vi "LoadGCSLowLevelVIs.vi"(11 "GCS Merged Drivers Low-Level Path":path) -> (3 "PI GCS Function\nReferences":T1)   [LabVIEW 2011]
uses:
  GCS_Interface.ctl
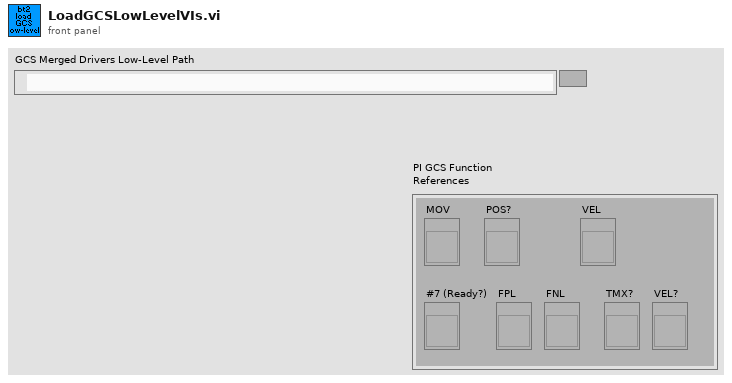
[diagram p1: front panel]
types:
  T1 = typedef "GCS_Interface.ctl" = cluster{"MOV":refnum<vi>, "VEL":refnum<vi>, "VEL?":refnum<vi>, "POS?":refnum<vi>, "TMX?":refnum<vi>, "#7 (Ready?)":refnum<vi>, "FPL":refnum<vi>, "FNL":refnum<vi>}
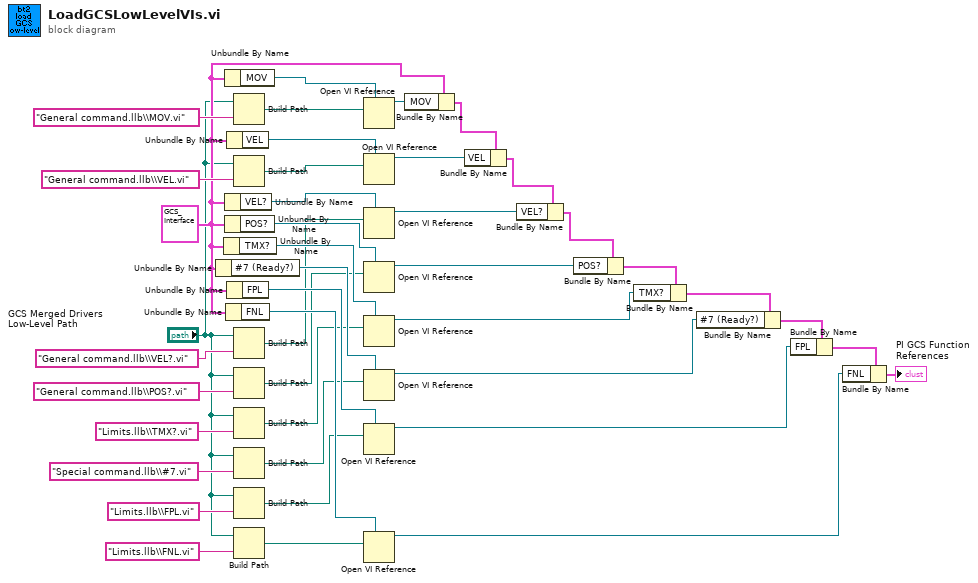
[diagram p0: block diagram]
diagram:
  w26 = T1 {"MOV"=refnum, "VEL"=refnum, "VEL?"=refnum, "POS?"=refnum, "TMX?"=refnum, "#7 (Ready?)"=refnum, "FPL"=refnum, "FNL"=refnum} ("PI GCS Function\nReferences")
  n1 = Unbundle By Name(w26) -> ("#7 (Ready?)"=w34:refnum<vi>)
  n2 = Unbundle By Name(w26) -> ("TMX?"=w37:refnum<vi>)
  n3 = Unbundle By Name(w26) -> ("MOV"=w33:refnum<vi>)
  n4 = Unbundle By Name(w26) -> ("VEL?"=w32:refnum<vi>)
  n5 = Unbundle By Name(w26) -> ("POS?"=w35:refnum<vi>)
  n6 = Unbundle By Name(w26) -> ("FNL"=w29:refnum<vi>)
  n7 = Unbundle By Name(w26) -> ("VEL"=w31:refnum<vi>)
  n8 = Unbundle By Name(w26) -> ("FPL"=w30:refnum<vi>)
  n9 = Build Path(base path="GCS Merged Drivers Low-Level Path", name or relative path="General command.llb\\MOV.vi") -> (appended path=w17:path)
  n10 = Build Path(base path="GCS Merged Drivers Low-Level Path", name or relative path="General command.llb\\VEL.vi") -> (appended path=w15:path)
  n11 = Build Path(base path="GCS Merged Drivers Low-Level Path", name or relative path="General command.llb\\VEL?.vi") -> (appended path=w12:path)
  n12 = Build Path(base path="GCS Merged Drivers Low-Level Path", name or relative path="General command.llb\\POS?.vi") -> (appended path=w27:path)
  n13 = Build Path(base path="GCS Merged Drivers Low-Level Path", name or relative path="Limits.llb\\TMX?.vi") -> (appended path=w10:path)
  n14 = Build Path(base path="GCS Merged Drivers Low-Level Path", name or relative path="Special command.llb\\#7.vi") -> (appended path=w5:path)
  n15 = Build Path(base path="GCS Merged Drivers Low-Level Path", name or relative path="Limits.llb\\FPL.vi") -> (appended path=w4:path)
  n16 = Build Path(base path="GCS Merged Drivers Low-Level Path", name or relative path="Limits.llb\\FNL.vi") -> (appended path=w1:path)
  n17 = Open VI Reference(type specifier VI Refnum (for type only)=w33, vi path=w17) -> (vi reference=w16:refnum<vi>)  [unwired: 4 in, 1 out]
  n18 = Open VI Reference(type specifier VI Refnum (for type only)=w31, vi path=w15) -> (vi reference=w14:refnum<vi>)  [unwired: 4 in, 1 out]
  n19 = Open VI Reference(type specifier VI Refnum (for type only)=w32, vi path=w12) -> (vi reference=w13:refnum<vi>)  [unwired: 4 in, 1 out]
  n20 = Open VI Reference(type specifier VI Refnum (for type only)=w35, vi path=w27) -> (vi reference=w11:refnum<vi>)  [unwired: 4 in, 1 out]
  n21 = Open VI Reference(type specifier VI Refnum (for type only)=w37, vi path=w10) -> (vi reference=w9:refnum<vi>)  [unwired: 4 in, 1 out]
  n22 = Open VI Reference(type specifier VI Refnum (for type only)=w34, vi path=w5) -> (vi reference=w8:refnum<vi>)  [unwired: 4 in, 1 out]
  n23 = Open VI Reference(type specifier VI Refnum (for type only)=w30, vi path=w4) -> (vi reference=w3:refnum<vi>)  [unwired: 4 in, 1 out]
  n24 = Open VI Reference(type specifier VI Refnum (for type only)=w29, vi path=w1) -> (vi reference=w2:refnum<vi>)  [unwired: 4 in, 1 out]
  n25 = Bundle By Name(cluster=w26, "MOV"=w16) -> (w25:T1)
  n26 = Bundle By Name(cluster=w25, "VEL"=w14) -> (w24:T1)
  n27 = Bundle By Name(cluster=w24, "VEL?"=w13) -> (w23:T1)
  n28 = Bundle By Name(cluster=w23, "POS?"=w11) -> (w22:T1)
  n29 = Bundle By Name(cluster=w22, "TMX?"=w9) -> (w21:T1)
  n30 = Bundle By Name(cluster=w21, "#7 (Ready?)"=w8) -> (w20:T1)
  n31 = Bundle By Name(cluster=w20, "FPL"=w3) -> (w19:T1)
  n32 = Bundle By Name(cluster=w19, "FNL"=w2) -> (→"PI GCS Function\nReferences":T1)
